vi "EXI-8000PCIe.vi"() -> ()   [LabVIEW 2020]
uses:
  <vilib>/Utility/miscctls.llb/LVPointTypeDef.ctl
  LabVIEW 2020 Toolkits/toolkits_lv2020_32bit/Synchronization.llb/SynchRefs_SetGet.ctl
  LabVIEW 2020 Toolkits/VI Server Toolkit/VI Server Libraries/VI Server Controls.llb/VI Server_Properties.ctl
  LabVIEW 2020 Toolkits/VI Server Toolkit/VI Server Libraries/VI Server_GetControl.llb/VI Server_STR_Get.vi
  LabVIEW 2020 Toolkits/VI Server Toolkit/VI Server Libraries/VI Server_Set Controls.llb/Set STR Control.vi
  LabVIEW 2020 Toolkits/VI Server Toolkit/VI Server Libraries/VI Server_SetControl.llb/VI Server_U16_Set.vi
  LabVIEW 2020 Toolkits/VI Server Toolkit/VI Server Libraries/VI Server_SetControl.llb/VI Server_BOOL_Set.vi
  LabVIEW 2020 Toolkits/VI Server Toolkit/VI Server Toolkit LV2013.lvlib
panel:
  out "System.Message":string caption="System Message"
  in  "Help":bool
  in  "FP.Hide":bool caption="FrontPanel.Hide"
  in  "EXIT":bool
  in  "Tab.Main":enum32{"1553 BC", "1553 RT", "SETTINGS"}(tab)
  in  "BC.DataWords.DisplayFormat":u16(ring) caption="Data Words: Display Format" items=["Decimal", "Hex"]
  in  "BC.SavedData.Selector":u16(ring) caption="Saved Data Selector" items=["New Data Set", "Data Set 1", "Data Set 2"]
  in  "BC.SaveData":bool
  in  "BC.Reset.DataWords":bool
  out "BC.Msg.Status.Loop.Counter":u16 caption="Msg. Status Loop Counter"
  out "BC.Msg.Returned.Flag":bool caption="Msg. Returned Flag"
  out "BC.Msg.Status":u16 caption="Msg. Status" format="%.0x"
  out "BC.TimeTag":u32 caption="Time Tag" format="%.0x"
  out "BC.Command.Word":u16 caption="Command Word" format="%.0x"
  in  "BC.MinFrameTime":i32=200 caption="Min Frame Time" min=100 format="%d usec"
  in  "BC.TimesToExecuteFrame":i32=1 caption="Times To Execute" min=1
  in  "BC.Message.Type":u16(ring)=1 caption="Message Type" items=["RT2BC"=0, "BC2RT"=1, "RT2RT"=2, "MODE"=3, "BRD_RCV"=4, "BRD_RT2RT"=5, "BRD_MODE"=6, "MINOR_FRAME"=15]
  in  "BC.RX/TX":u16(ring) caption="RX/TX" items=["RECEIVE", "TRANSMIT"]
  in  "BC.Word.Count":i32 caption="Word Count" max=32
  in  "BC.RT.Subaddress":i32 caption="RT Subaddress" max=31
  in  "BC.RT.Number":i32 caption="RT Number" max=31
  in  "BC.Buss.Selector":u16(ring) caption="Buss Selector" items=["Bus A", "Bus B"]
  in  "BC.Start":bool
  out "BC.Init.Mode":i32(ring)=4 caption="Mode" items=["RT"=2, "BC/CONCURRENT RT"=4, "MONITOR - BLOCK"=8, "MONITOR - LOOKUP"=32, "LL 0018"=68]
  out "BC.FW.Revision":i32=161 caption="FW Revision"
  out "BC.Module.ID":i32=69 caption="Module ID"
  out "BC.Board.Status.Flags":string[](array[string])=["BOARD_READY", "RAM_OK", "TIMERS_OK", "SELF_TEST_OK", "BOARD_HALTED", "PX_BOARD"] caption="Board Status Flags"
  out "BC.CardInitialized":bool caption="Card Initialized"
  in  "BC.Mode":u16(ring)=4 caption="Mode" items=["RT"=2, "BC/CONCURRENT RT"=4, "MONITOR - BLOCK"=8, "MONITOR - LOOKUP"=32, "LL 0018"=68]
  in  "BC.Module":u16 caption="Module"
  in  "BC.Device":u16 caption="Device" max=255 step=1
  in  "BC.DW-32":u16 caption="DW-32" format="%04x"
  in  "BC.DW-24":u16 caption="DW-24" format="%04x"
  in  "BC.DW-16":u16 caption="DW-16" format="%04x"
  in  "BC.DW-8":u16 caption="DW-08" format="%04x"
  in  "BC.DW-31":u16 caption="DW-31" format="%04x"
  in  "BC.DW-23":u16 caption="DW-23" format="%04x"
  in  "BC.DW-15":u16 caption="DW-15" format="%04x"
  in  "BC.DW-7":u16 caption="DW-07" format="%04x"
  in  "BC.DW-30":u16 caption="DW-30" format="%04x"
  in  "BC.DW-22":u16 caption="DW-22" format="%04x"
  in  "BC.DW-14":u16 caption="DW-14" format="%04x"
  in  "BC.DW-6":u16 caption="DW-06" format="%04x"
  in  "BC.DW-29":u16 caption="DW-29" format="%04x"
  in  "BC.DW-21":u16 caption="DW-21" format="%04x"
  in  "BC.DW-13":u16 caption="DW-13" format="%04x"
  in  "BC.DW-5":u16 caption="DW-05" format="%04x"
  in  "BC.DW-28":u16 caption="DW-28" format="%04x"
  in  "BC.DW-20":u16 caption="DW-20" format="%04x"
  in  "BC.DW-12":u16 caption="DW-12" format="%04x"
  in  "BC.DW-4":u16 caption="DW-04" format="%04x"
  in  "BC.DW-25":u16 caption="DW-25" format="%04x"
  in  "BC.DW-17":u16 caption="DW-17" format="%04x"
  in  "BC.DW-9":u16 caption="DW-09" format="%04x"
  in  "BC.DW-1":u16 caption="DW-01" format="%04x"
  in  "BC.DW-26":u16 caption="DW-26" format="%04x"
  in  "BC.DW-18":u16 caption="DW-18" format="%04x"
  in  "BC.DW-10":u16 caption="DW-10" format="%04x"
  in  "BC.DW-2":u16 caption="DW-02" format="%04x"
  in  "BC.DW-27":u16 caption="DW-27" format="%04x"
  in  "BC.DW-19":u16 caption="DW-19" format="%04x"
  in  "BC.DW-11":u16 caption="DW-11" format="%04x"
  in  "BC.DW-3":u16 caption="DW-03" format="%04x"
  in  "RT.SavedData.ReLoad":bool
  in  "RT.SavedData.Selector":u16(ring) caption="Saved Data Selector" items=["New Data Set", "Data Set 1"]
  in  "RT.SaveData":bool
  in  "RT.DataWords.DisplayFormat":u16(ring) caption="Data Words: Display Format" items=["Decimal", "Hex"]
  in  "RT.Reset.Data":bool
  out "RT.Message":string[][](table) caption="Message box"
  in  "RT.Blk.Update":bool caption="Block Update"
  in  "RT.Blk.Number":i32=1 caption="Block Number" min=1 max=31
  in  "RT.RX/TX":u16(ring) caption="RX/TX" items=["RECEIVE", "TRANSMIT"]
  in  "RT.Subaddress":i32 caption="RT Subaddress" max=31
  in  "RT.Number":i32 caption="RT Number" max=31
  out "RT.Init.Mode":i32(ring)=4 caption="Mode" items=["MODE NOT CONFIGURED"=0, "RT"=2, "BC/CONCURRENT RT"=4, "MONITOR - BLOCK"=8, "MONITOR - LOOKUP"=32, "LL 0018"=68]
  out "RT.FW.Revision":i32=161 caption="FW Revision"
  out "RT.Module.ID":i32=69 caption="Module ID"
  out "RT.Board.Status.Flags":string[](array[string])=["BOARD_READY", "RAM_OK", "TIMERS_OK", "SELF_TEST_OK", "BOARD_HALTED", "PX_BOARD"] caption="Board Status Flags"
  out "RT.CardInitialized":bool caption="Card Initialized"
  in  "RT.Start":bool
  in  "RT.Mode":u16(ring)=4 caption="Mode" items=["RT"=2, "BC/CONCURRENT RT"=4, "MONITOR - BLOCK"=8, "MONITOR - LOOKUP"=32, "LL 0018"=68]
  in  "RT.Module":u16 caption="Module"
  in  "RT.Device":u16 caption="Device" max=255 step=1
  out "RT.Msg.Returned.Flag":bool caption="Msg. Returned Flag"
  in  "RT.DW-32":u16 caption="DW-32" format="%04x"
  in  "RT.DW-24":u16 caption="DW-24" format="%04x"
  in  "RT.DW-16":u16 caption="DW-16" format="%04x"
  in  "RT.DW-8":u16 caption="DW-08" format="%04x"
  in  "RT.DW-31":u16 caption="DW-31" format="%04x"
  in  "RT.DW-23":u16 caption="DW-23" format="%04x"
  in  "RT.DW-15":u16 caption="DW-15" format="%04x"
  in  "RT.DW-7":u16 caption="DW-07" format="%04x"
  in  "RT.DW-30":u16 caption="DW-30" format="%04x"
  in  "RT.DW-22":u16 caption="DW-22" format="%04x"
  in  "RT.DW-14":u16 caption="DW-14" format="%04x"
  in  "RT.DW-6":u16 caption="DW-06" format="%04x"
  in  "RT.DW-29":u16 caption="DW-29" format="%04x"
  in  "RT.DW-21":u16 caption="DW-21" format="%04x"
  in  "RT.DW-13":u16 caption="DW-13" format="%04x"
  in  "RT.DW-5":u16 caption="DW-05" format="%04x"
  in  "RT.DW-28":u16 caption="DW-28" format="%04x"
  in  "RT.DW-20":u16 caption="DW-20" format="%04x"
  in  "RT.DW-12":u16 caption="DW-12" format="%04x"
  in  "RT.DW-4":u16 caption="DW-04" format="%04x"
  in  "RT.DW-25":u16 caption="DW-25" format="%04x"
  in  "RT.DW-17":u16 caption="DW-17" format="%04x"
  in  "RT.DW-9":u16 caption="DW-09" format="%04x"
  in  "RT.DW-1":u16 caption="DW-01" format="%04x"
  in  "RT.DW-26":u16 caption="DW-26" format="%04x"
  in  "RT.DW-18":u16 caption="DW-18" format="%04x"
  in  "RT.DW-10":u16 caption="DW-10" format="%04x"
  in  "RT.DW-2":u16 caption="DW-02" format="%04x"
  in  "RT.DW-27":u16 caption="DW-27" format="%04x"
  in  "RT.DW-19":u16 caption="DW-19" format="%04x"
  in  "RT.DW-11":u16 caption="DW-11" format="%04x"
  in  "RT.DW-3":u16 caption="DW-03" format="%04x"
  out "Instr.Responce":string caption="Instrument Responce"
  out "Instr.Command.Sent":string caption="Command: Sent"
  in  "UDP.Test.String2.Send":bool
  in  "UDP.Test.String2":string caption="UDP: Test String 2"
  in  "UDP.Port.Receiver":u16=58433 caption="UDP: Port.Receiver"
  in  "UDP.Port.Read":u16=58432 caption="UDP: Port.Read"
  in  "UDP.LocalPort.Write":u16=58434 caption="UDP: Local Port.Write"
  in  "UDP.IP.Address":string="234.5.6.7" caption="UDP: IP Address"
  in  "UDP.Test.String1.Send":bool
  in  "UDP.Test.String1":string caption="UDP: Test String 1"
  in  "UDP.Responce.String.Monitor":bool
  out "UDP.ExecEng.Message.String":string caption="UDP: Execution Engine Message String"
  out "error out":errorcluster={"status"=TRUE, "code"=1055, "source"="Property Node in VI Server Toolkit LV2013.lvlib:VI server_Set Control Value from String Format.vi:5200001->DMM6500_UDP_ExecEng_Instruction_APPLY.vi->DMM6500_UDP_MAIN.vi->Keithley2100.vi"}
  in  "error in":errorcluster
  # "NOTES:\n\n1. To request data from RT the\n\"Format Message\" /Transmit/Receive\nshould be set to \"Transmit\".\nThe Message Type should be set to\n\"RT2BC.\nData Words shall be empty array.\nIf the Status Word = x8201, the BC\n module did not receive data."
  # "Multicast IP addresses must be in the 224.0.0.0 to 239.255.255.255 range."
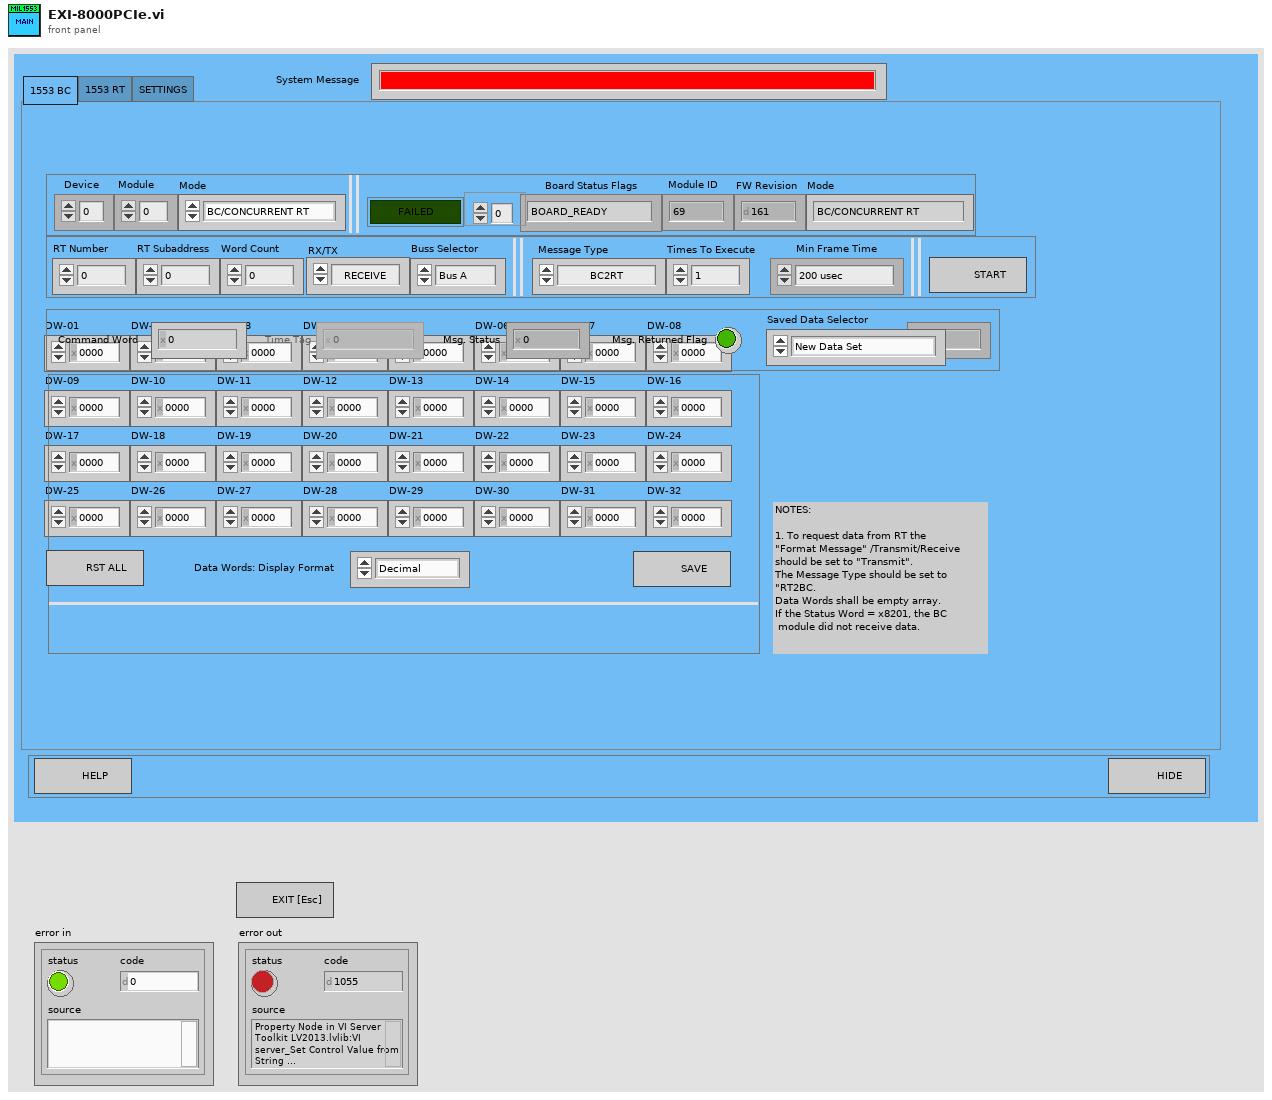
[diagram p1: front panel]
types:
  T1 = typedef "LVPointTypeDef.ctl" = cluster{"Horizontal":i16, "Vertical":i16}
  T2 = typedef "VI Server_RefsCluster.ctl" = cluster{"Labels":string[], "Refs":refnum<vi>[], "VI Ref":refnum<vi>}
  T3 = typedef "SynchRefs_SetGet.ctl" = enum16{"Set", "Get"}
  T4 = enum8{"Enabled", "Disabled", "Disabled and Grayed Out"}
  T5 = typedef "VI Server Toolkit LV2013.lvlib/VI Server_Properties.ctl" = string
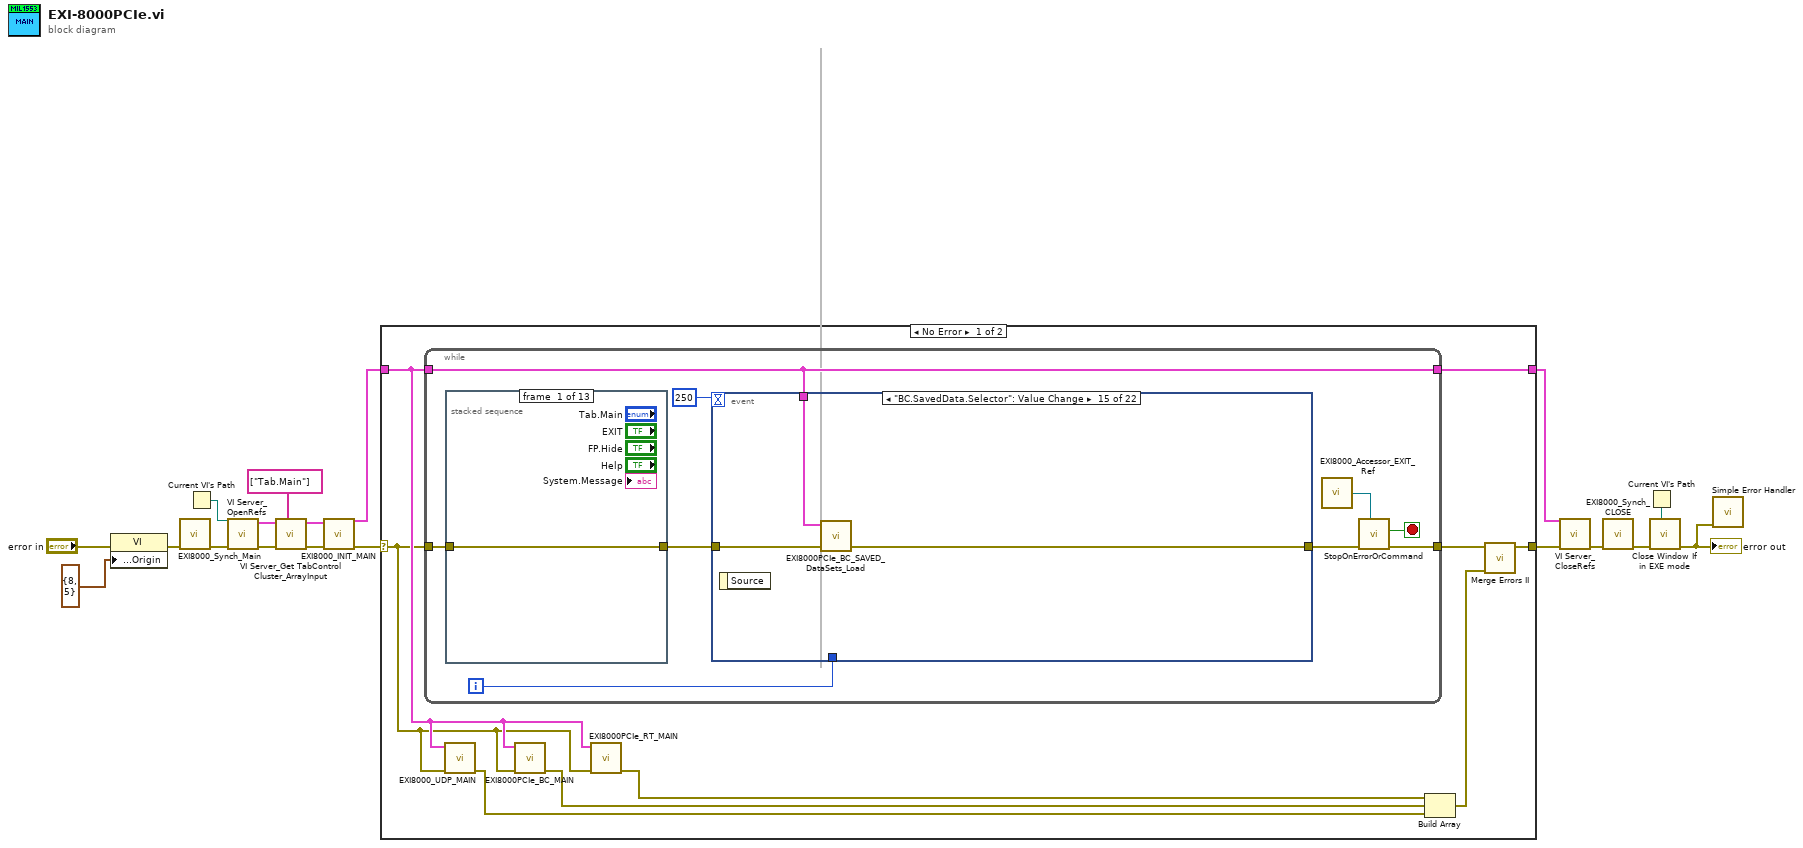
[diagram p0: block diagram]
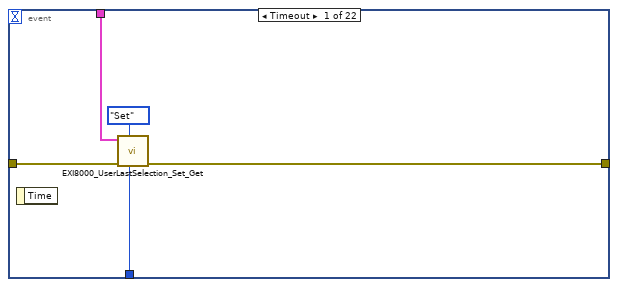
[diagram p2: hidden frame]
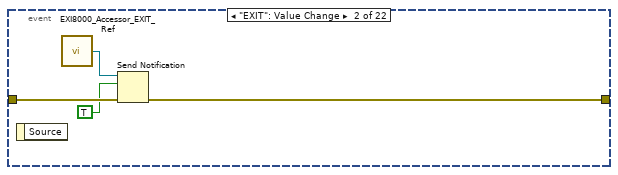
[diagram p3: hidden frame]
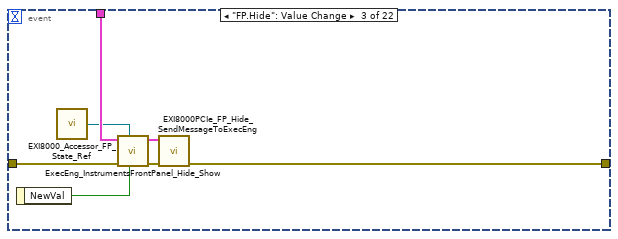
[diagram p4: hidden frame]
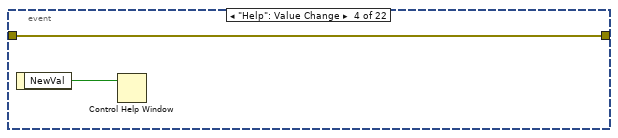
[diagram p5: hidden frame]
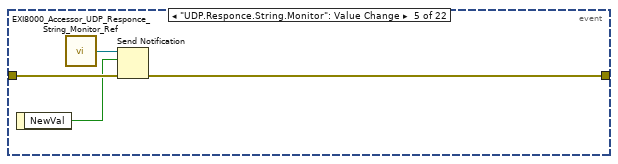
[diagram p6: hidden frame]
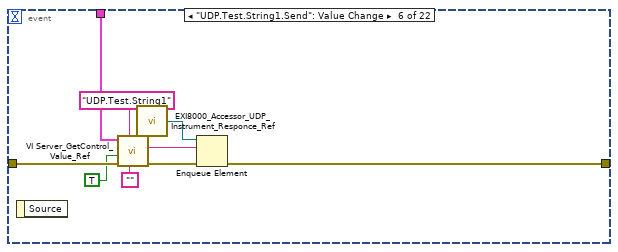
[diagram p7: hidden frame]
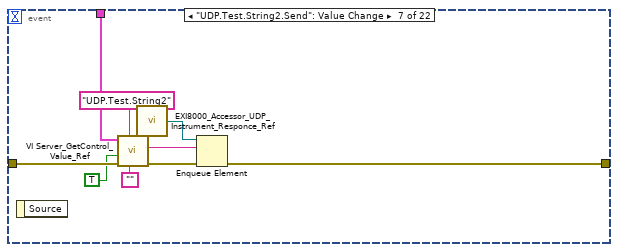
[diagram p8: hidden frame]
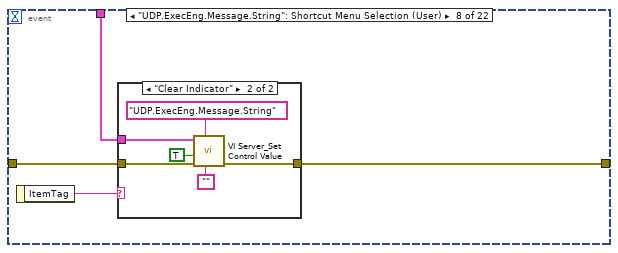
[diagram p9: hidden frame]
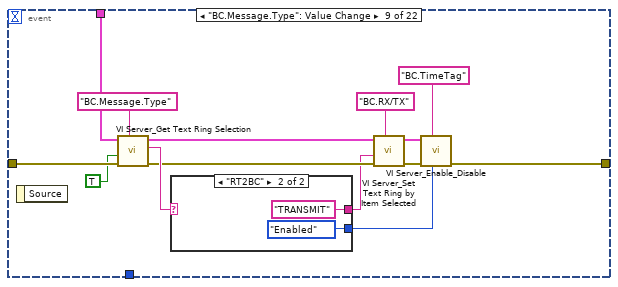
[diagram p11: hidden frame]
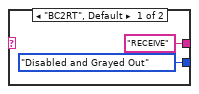
[diagram p12: hidden frame]
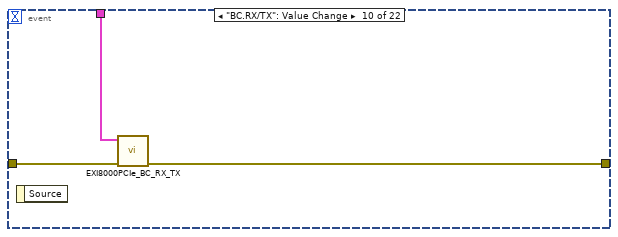
[diagram p13: hidden frame]
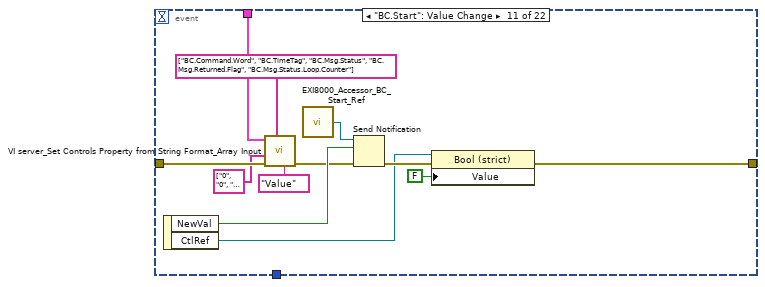
[diagram p14: hidden frame]
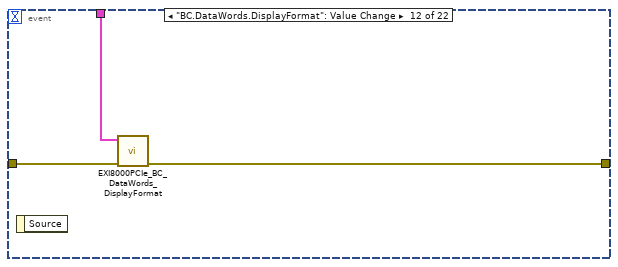
[diagram p15: hidden frame]
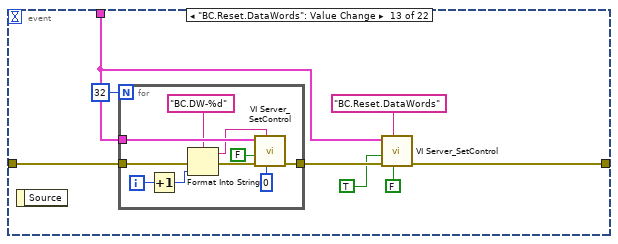
[diagram p16: hidden frame]
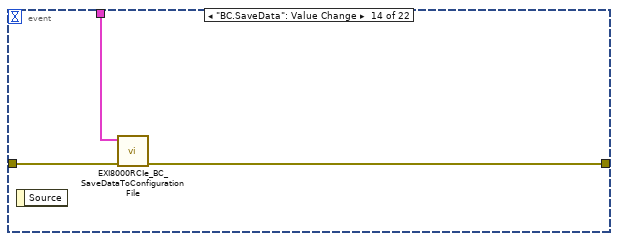
[diagram p17: hidden frame]
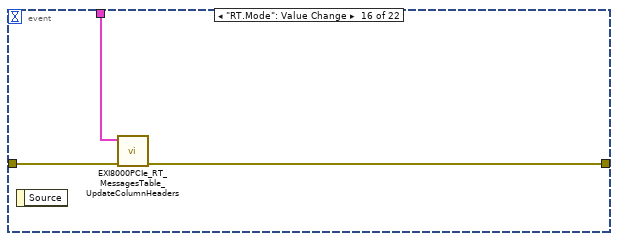
[diagram p18: hidden frame]
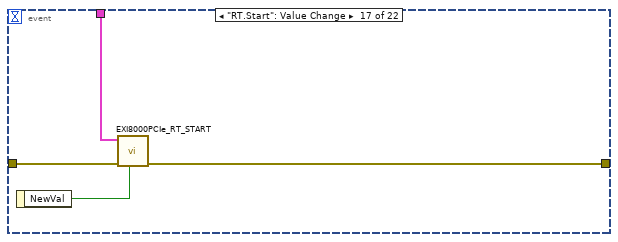
[diagram p19: hidden frame]
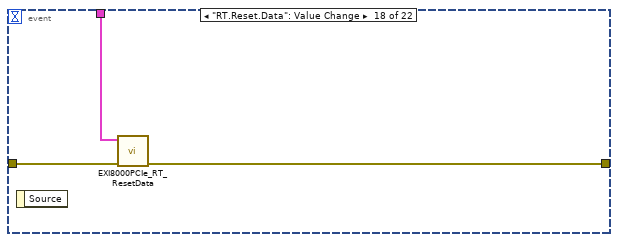
[diagram p20: hidden frame]
diagram:
  n1 = property class="VI"(error in="error in", "Front Panel Window:Origin"=T1 {"Horizontal"=8, "Vertical"=5}) -> (error out=w12:errorcluster)  [unwired: 1 in, 1 out]
  n2 = call "EXI8000_Synch_Main.vi"("error in"=w12) -> ("error out"=w13:errorcluster)  [unwired: 10 in]
  n3 = Current VI's Path() -> (path=w17:path)
  n4 = call "VI Server_OpenRefs.vi"("error in"=w13, "VI Path"=w17) -> ("error out"=w14:errorcluster, "VI Server.RefsCluster"=w15:T2)  [unwired: 8 in]
  n5 = call "VI Server_Get TabControl Cluster_ArrayInput.vi"("TabControl Labels[]"=string[] ["Tab.Main"], "error in"=w14, "VI Server Cluster"=w15) -> ("error out"=w11:errorcluster, "VI Server Cluster.OUT"=w10:T2)  [unwired: 7 in]
  n6 = call "EXI8000_INIT_MAIN.vi"("error in (no error)"=w11, "VI Server Cluster"=w10) -> ("error out"=w9:errorcluster, "VI Server Cluster DUP"=w8:T2)  [unwired: 8 in]
  n7 = case shown="No Error" w9 {
    selector: w9 -> [w20 w172]
    tunnel: [w24 w172] -> w7
    tunnel: w8 -> [w21 w171]
    tunnel: [w27 w171] -> w6
    frame No Error {
      n8 = while {
        tunnel: w20 -> [w36]
        tunnel: [w30] -> w25
        tunnel: w21 -> [w32]
        tunnel: [w32] -> w27
        i -> [w33]
        stop <- w29 stop-if-true
        n9 = stacked-sequence {
          tunnel: w36 -> [w170 _ _ _ _ _ _ _ _ _ _ _ _]
          tunnel: [w170 _ _ _ _ _ _ _ _ _ _ _ _] -> w35
          frame #0 {
          }
          frame #1 {
          }
          frame #2 {
          }
          frame #3 {
          }
          frame #4 {
          }
          frame #5 {
          }
          frame #6 {
          }
          frame #7 {
          }
          frame #8 {
          }
          frame #9 {
          }
          frame #10 {
          }
          frame #11 {
          }
          frame #12 {
          }
        }
        n10 = event shown="[14] \"BC.SavedData.Selector\": Value Change" {
          selector: _ -> [_ _ _ _ _ _ _ _ _ _ _ _ _ _ _ _ _ _ _ _ _ _]
          dyn-events: _ -> [_ _ _ _ _ _ _ _ _ _ _ _ _ _ _ _ _ _ _ _ _ _]
          timeout: 250 -> [_ _ _ _ _ _ _ _ _ _ _ _ _ _ _ _ _ _ _ _ _ _]
          tunnel: w35 -> [w40 w45 w51 w54 w58 w67 w76 w80 w101 w108 w117 w121 w131 w142 w147 w150 w152 w155 w160 w163 w166 w167]
          tunnel: w33 -> [w39 _ _ _ _ _ _ _ _ _ _ _ _ _ _ _ _ _ _ _ _ _]
          tunnel: [w38 w43 w52 w54 w56 w65 w74 w78 w91 w106 w111 w122 w128 w143 w146 w148 w154 w156 w158 w162 w164 w168] -> w31
          tunnel: w32 -> [w37 _ w49 _ _ w64 w73 w77 w100 w107 w116 w123 w127 w144 w145 w149 w153 w157 w159 w161 w165 w169]
          event Timeout {
            n11 = event-data() -> ()  [unwired: 1 in, 1 out]
            n12 = call "EXI8000_UserLastSelection_Set_Get.vi"("LoopCounter"=w39, "SynchRefs.Set/Get"=SynchRefs_SetGet."Set", "error in"=w40, "VI Server.RefsCluster"=w37) -> ("error out"=w38:errorcluster)  [unwired: 6 in, 1 out]
          }
          event "EXIT": Value Change {
            n13 = event-data() -> ()  [unwired: 1 in, 1 out]
            n14 = call "EXI8000_Accessor_EXIT_Ref.vi"() -> ("EXIT"=w44:refnum<notifier>)  [unwired: 6 in]
            n15 = Send Notification(notification=TRUE, notifier=w44, error in (no error)=w45) -> (error out=w43:errorcluster)  [unwired: 1 out]
          }
          event "FP.Hide": Value Change {
            n16 = event-data() -> ("NewVal"=w48:bool)  [unwired: 1 in]
            n17 = call "EXI8000_Accessor_FP_State_Ref.vi"() -> ("FP.State"=w46:refnum<notifier>)  [unwired: 6 in]
            n18 = call "ExecEng_InstrumentsFrontPanel_Hide_Show.vi"("FP.Hide/Show"=w48, "FP.State"=w46, "error in (no error)"=w51, "VI Server Cluster"=w49) -> ("error out"=w47:errorcluster, "VI Server Cluster DUP"=w50:T2)  [unwired: 6 in]
            n19 = call "EXI8000PCIe_FP_Hide_SendMessageToExecEng.vi"("error in (no error)"=w47, "VI Server Cluster"=w50) -> ("error out"=w52:errorcluster)  [unwired: 9 in]
          }
          event "Help": Value Change {
            n20 = event-data() -> ("NewVal"=w53:bool)  [unwired: 1 in]
            n21 = Control Help Window(1:w53) -> ()  [unwired: 1 in]
          }
          event "UDP.Responce.String.Monitor": Value Change {
            n22 = event-data() -> ("NewVal"=w55:bool)  [unwired: 1 in]
            n23 = call "EXI8000_Accessor_UDP_Responce_String_Monitor_Ref.vi"() -> ("UDP.ExecEng.Command.String.Monitor"=w57:refnum<notifier>)  [unwired: 6 in]
            n24 = Send Notification(notification=w55, notifier=w57, error in (no error)=w58) -> (error out=w56:errorcluster)  [unwired: 1 out]
          }
          event "UDP.Test.String1.Send": Value Change {
            n25 = event-data() -> ()  [unwired: 1 in, 1 out]
            n26 = call-poly "VI Server_GetControl_Value_Ref.vi"("DataType"="", "Control.Label"="UDP.Test.String1", "error in"=w67, "SingleInstance"=TRUE, "VI Server.RefsCluster"=w64) -> ("error out"=w66:errorcluster, "Value"=w59:string)  [unwired: 3 in, 2 out]
            n27 = call "EXI8000_Accessor_UDP_Instrument_Responce_Ref.vi"() -> ("UDP.Instrument.Responce.Q"=w60:refnum<queue>)  [unwired: 6 in]
            n28 = Enqueue Element(queue=w60, element=w59, error in (no error)=w66) -> (error out=w65:errorcluster)  [unwired: 1 in, 2 out]
          }
          event "UDP.Test.String2.Send": Value Change {
            n29 = event-data() -> ()  [unwired: 1 in, 1 out]
            n30 = call-poly "VI Server_GetControl_Value_Ref.vi"("DataType"="", "Control.Label"="UDP.Test.String2", "error in"=w76, "SingleInstance"=TRUE, "VI Server.RefsCluster"=w73) -> ("error out"=w75:errorcluster, "Value"=w68:string)  [unwired: 3 in, 2 out]
            n31 = call "EXI8000_Accessor_UDP_Instrument_Responce_Ref.vi"() -> ("UDP.Instrument.Responce.Q"=w69:refnum<queue>)  [unwired: 6 in]
            n32 = Enqueue Element(queue=w69, element=w68, error in (no error)=w75) -> (error out=w74:errorcluster)  [unwired: 1 in, 2 out]
          }
          event "UDP.ExecEng.Message.String": Shortcut Menu Selection (User) {
            n33 = event-data() -> ("ItemTag"=w79:string)  [unwired: 1 in]
            n34 = case shown="\"Clear Indicator\"" w79 {
              tunnel: w80 -> [w81 w87]
              tunnel: [w81 w86] -> w78
              tunnel: w77 -> [_ w85]
              frame "", Default {
              }
              frame "Clear Indicator" {
                n35 = call-poly "VI Server_Set Control Value.vi"("New Value"="", "Label"="UDP.ExecEng.Message.String" ("Control.Label"), "error in"=w87, "Single Instance (T)"=TRUE ("SingleInstance"), "VI Server Cluster"=w85) -> ("error out"=w86:errorcluster)  [unwired: 4 in, 2 out]
              }
            }
          }
          event "BC.Message.Type": Value Change {
            n36 = event-data() -> ()  [unwired: 1 in, 1 out]
            n37 = call "VI Server_Get Text Ring Selection.vi"("Label"="BC.Message.Type", "error in"=w101, "Single Instance (T)"=TRUE, "VI Server Cluster"=w100) -> ("error out"=w96:errorcluster, "Selection"=w97:string, "VI Server Custer.DUP"=w93:T2)  [unwired: 2 in, 3 out]
            n38 = case shown="\"RT2BC\"" w97 {
              tunnel: ["RECEIVE" "TRANSMIT"] -> w95
              tunnel: [T4."Disabled and Grayed Out" ("Disabled") T4."Enabled" ("Disabled")] -> w88
              frame "BC2RT", Default {
              }
              frame "RT2BC" {
              }
            }
            n39 = call "VI Server_Set Text Ring by Item Selected.vi"("Label"="BC.RX/TX", "error in"=w96, "Item"=w95, "VI Server.RefsCluster"=w93) -> ("error out"=w92:errorcluster, "VI Server Cluster.DUP"=w90:T2)  [unwired: 5 in, 1 out]
            n40 = call "VI Server_Enable_Disable.vi"("Disabled"=w88, "Label"="BC.TimeTag", "error in"=w92, "VI Server Cluster"=w90) -> ("error out"=w91:errorcluster)  [unwired: 5 in, 2 out]
          }
          event "BC.RX/TX": Value Change {
            n41 = event-data() -> ()  [unwired: 1 in, 1 out]
            n42 = call "EXI8000PCIe_BC_RX_TX.vi"("error in (no error)"=w108, "VI Server Cluster"=w107) -> ("error out"=w106:errorcluster)  [unwired: 8 in, 1 out]
          }
          event "BC.Start": Value Change {
            n43 = event-data() -> ("NewVal"=w119:bool, "CtlRef"=w110:refnum<vi>)  [unwired: 1 in]
            n44 = call "VI server_Set Controls Property from String Format_Array Input.vi"("Property"=T5 "Value", "Labels"=string[] ["BC.Command.Word", "BC.TimeTag", "BC.Msg.Status", "BC.Msg.Returned.Flag", "BC.Msg.Status.Loop.Counter"], "error in (no error)"=w117, "Values"=string[] ["0", "0", "0", "0", "0"], "VI Server.RefsCluster"=w116) -> ("error out"=w118:errorcluster)  [unwired: 5 in, 1 out]
            n45 = call "EXI8000_Accessor_BC_Start_Ref.vi"() -> ("BC.Start"=w120:refnum<notifier>)  [unwired: 6 in]
            n46 = Send Notification(notification=w119, notifier=w120, error in (no error)=w118) -> (error out=w112:errorcluster)  [unwired: 1 out]
            n47 = property class="Bool (strict)"(reference=w110, error in=w112, "Value"=FALSE) -> (error out=w111:errorcluster)  [unwired: 1 out]
          }
          event "BC.DataWords.DisplayFormat": Value Change {
            n48 = event-data() -> ()  [unwired: 1 in, 1 out]
            n49 = call "EXI8000PCIe_BC_DataWords_DisplayFormat.vi"("error in (no error)"=w121, "VI Server Cluster"=w123) -> ("error out"=w122:errorcluster)  [unwired: 8 in, 1 out]
          }
          event "BC.Reset.DataWords": Value Change {
            n50 = event-data() -> ()  [unwired: 1 in, 1 out]
            n51 = for {
              N: 32 -> [_]
              tunnel: w127 -> [w140]
              tunnel: w131 -> [w138]
              tunnel: [w141] -> w129
              i -> [w135]
              n52 = Increment(x=w135) -> (x+1=w134:i32)
              n53 = Format Into String(format string="BC.DW-%d", error in=w138, w134) -> (resulting string=w132:string, error out=w137:errorcluster)  [unwired: 1 in]
              n54 = call-poly "VI Server_SetControl.vi"("Data"=u16 0, "Control.Label"=w132, "error in"=w137, "SingleInstance"=FALSE, "VI Server.RefsCluster"=w140) -> ("error out"=w141:errorcluster)  [unwired: 4 in, 2 out]
            }
            n55 = call-poly "VI Server_SetControl.vi"("Data"=FALSE, "Control.Label"="BC.Reset.DataWords", "error in"=w129, "SingleInstance"=TRUE, "VI Server.RefsCluster"=w127) -> ("error out"=w128:errorcluster)  [unwired: 4 in, 2 out]
          }
          event "BC.SaveData": Value Change {
            n56 = event-data() -> ()  [unwired: 1 in, 1 out]
            n57 = call "EXI8000RCIe_BC_SaveDataToConfigurationFile.vi"("error in (no error)"=w142, "VI Server Cluster"=w144) -> ("error out"=w143:errorcluster)  [unwired: 9 in]
          }
          event "BC.SavedData.Selector": Value Change {
            n58 = event-data() -> ()  [unwired: 1 in, 1 out]
            n59 = call "EXI8000PCIe_BC_SAVED_DataSets_Load.vi"("error in (no error)"=w147, "VI Server Cluster"=w145) -> ("error out"=w146:errorcluster)  [unwired: 9 in]
          }
          event "RT.Mode": Value Change {
            n60 = event-data() -> ()  [unwired: 1 in, 1 out]
            n61 = call "EXI8000PCIe_RT_MessagesTable_UpdateColumnHeaders.vi"("error in (no error)"=w150, "VI Server Cluster"=w149) -> ("error out"=w148:errorcluster)  [unwired: 8 in, 1 out]
          }
          event "RT.Start": Value Change {
            n62 = event-data() -> ("NewVal"=w151:bool)  [unwired: 1 in]
            n63 = call "EXI8000PCIe_RT_START.vi"("RT.Start"=w151, "error in (no error)"=w152, "VI Server Cluster"=w153) -> ("error out"=w154:errorcluster)  [unwired: 8 in]
          }
          event "RT.Reset.Data": Value Change {
            n64 = event-data() -> ()  [unwired: 1 in, 1 out]
            n65 = call "EXI8000PCIe_RT_ResetData.vi"("error in (no error)"=w155, "VI Server Cluster"=w157) -> ("error out"=w156:errorcluster)  [unwired: 8 in, 1 out]
          }
          event "RT.DataWords.DisplayFormat": Value Change {
            n66 = event-data() -> ()  [unwired: 1 in, 1 out]
            n67 = call "EXI8000PCIe_RT_DataWords_DisplayFormat.vi"("error in (no error)"=w160, "VI Server Cluster"=w159) -> ("error out"=w158:errorcluster)  [unwired: 8 in, 1 out]
          }
          event "RT.SaveData": Value Change {
            n68 = event-data() -> ()  [unwired: 1 in, 1 out]
            n69 = call "EXI8000RCIe_RT_SaveDataToConfigurationFile.vi"("error in (no error)"=w163, "VI Server Cluster"=w161) -> ("error out"=w162:errorcluster)  [unwired: 9 in]
          }
          event "RT.SavedData.Selector", "RT.SavedData.ReLoad": Value Change {
            n70 = event-data() -> ()  [unwired: 1 in, 1 out]
            n71 = call "EXI8000PCIe_RT_SAVED_DataSets_Load.vi"("error in (no error)"=w166, "VI Server Cluster"=w165) -> ("error out"=w164:errorcluster)  [unwired: 9 in]
          }
          event "RT.Blk.Update": Value Change {
            n72 = event-data() -> ()  [unwired: 1 in, 1 out]
            n73 = call "EXI8000PCIe_RT_UpdateDataBlock.vi"("error in (no error)"=w167, "VI Server Cluster"=w169) -> ("error out"=w168:errorcluster)  [unwired: 9 in]
          }
        }
        n74 = call "EXI8000_Accessor_EXIT_Ref.vi"() -> ("EXIT"=w28:refnum<notifier>)  [unwired: 6 in]
        n75 = call "StopOnErrorOrCommand.vi"("STOP"=w28, "error in (no error)"=w31) -> ("error out"=w30:errorcluster, "STOP"=w29:bool)  [unwired: 8 in]
      }
      n76 = call "EXI8000_UDP_MAIN.vi"("error in (no error)"=w20, "VI Server.RefsCluster"=w21) -> ("error out"=w26:errorcluster)  [unwired: 9 in]
      n77 = call "EXI8000PCIe_BC_MAIN.vi"("error in"=w20, "VI Server.RefsCluster"=w21) -> ("error out"=w22:errorcluster)  [unwired: 9 in]
      n78 = call "EXI8000PCIe_RT_MAIN.vi"("error in"=w20, "VI Server.RefsCluster"=w21) -> ("error out"=w19:errorcluster)  [unwired: 9 in]
      n79 = Build Array(w19, w22, w26) -> (w23:errorcluster[])
      n80 = call "Merge Errors II.vi"("error array in"=w23, "error in 1 (no error)"=w25) -> ("error out.DUP"=w24:errorcluster)  [unwired: 4 in, 1 out]
    }
    frame Error {
    }
  }
  n81 = call "VI Server_CloseRefs.vi"("error in"=w7, "VI Server.RefsCluster"=w6) -> ("error out"=w5:errorcluster)  [unwired: 9 in]
  n82 = call "EXI8000_Synch_CLOSE.vi"("error in"=w5) -> ("error out"=w3:errorcluster)  [unwired: 10 in]
  n83 = Current VI's Path() -> (path=w2:path)
  n84 = call "Close Window If in EXE mode.vi"("TopLevelVI Path"=w2, "error in"=w3) -> ("error out"=w1:errorcluster)  [unwired: 9 in]
  "error out" <- w1
  n85 = call <vilib>:"Simple Error Handler.vi"("error in (no error)"=w1) -> ()  [unwired: 4 in, 5 out]
